vi "OpenArmSpikeMotors.vi"(10 "Name":string) -> ()   [LabVIEW 2013]
uses:
  <vilib>/Rock Robotics/SystemInterfaces/Typedef/FPGA_TypedefDigitalModule.ctl
  <vilib>/Rock Robotics/SystemInterfaces/DIO/FPGA_DIORelayChannel.ctl
  <vilib>/Rock Robotics/WPI/Relay/WPI_RelayDirection.ctl
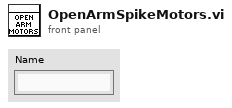
[diagram p1: front panel]
types:
  T1 = typedef "WPI_RelayDirection.ctl" = enum16{"Both directions", "Forward only", "Reverse only"}
  T2 = typedef "FPGA_DIORelayChannel.ctl" = enum8{"Relay 1", "Relay 2", "Relay 3", "Relay 4", "Relay 5", "Relay 6", "Relay 7", "Relay 8", "Invalid"}
  T3 = typedef "FPGA_TypedefDigitalModule.ctl" = enum16{"Digital Module 1", "Digital Module 2"}
  T4 = typedef "WPI_RelayDevRef.ctl" = cluster{"DevStatus":errorcluster, "Relay Channel":T2, "Digital Module":T3, "Relay Direction":T1}
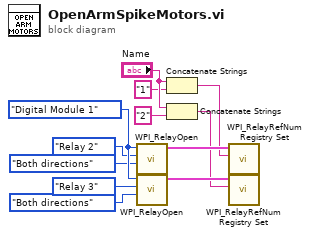
[diagram p0: block diagram]
diagram:
  w9 = FPGA_TypedefDigitalModule."Digital Module 1" ("Digital Module (Module 1)")
  n1 = call <vilib>:"WPI_RelayOpen.vi"("Relay Direction"=WPI_RelayDirection."Both directions", "Relay Channel"=FPGA_DIORelayChannel."Relay 2", "Digital Module (Module 1)"=w9) -> ("RelayDevRef"=w4:T4)  [unwired: 7 in, 1 out]
  n2 = call <vilib>:"WPI_RelayOpen.vi"("Relay Direction"=WPI_RelayDirection."Both directions", "Relay Channel"=FPGA_DIORelayChannel."Relay 3", "Digital Module (Module 1)"=w9) -> ("RelayDevRef"=w3:T4)  [unwired: 7 in, 1 out]
  n3 = Concatenate Strings("Name", "1") -> (w2:string)
  n4 = Concatenate Strings("Name", "2") -> (w1:string)
  n5 = call <vilib>:"WPI_RelayRefNum Registry Set.vi"("refnum name"=w2, "RelayDevRef"=w4) -> ()  [unwired: 8 in, 2 out]
  n6 = call <vilib>:"WPI_RelayRefNum Registry Set.vi"("refnum name"=w1, "RelayDevRef"=w3) -> ()  [unwired: 8 in, 2 out]
